vi "Execute.vi"(8 "error in (no error)":errorcluster, 10 "System In":refnum<class "abs_System.lvclass">, 11 "Node in":refnum<class "Set Boolean.lvclass">) -> (0 "error out":errorcluster, 1 "Status":T1, 2 "System Out":refnum<class "abs_System.lvclass">, 3 "Node out":refnum<class "Set Boolean.lvclass">)   [LabVIEW 2021, in "BT.lvlib" / "Set Boolean.lvclass"]
uses:
  Set Boolean.lvclass
  C:/Users/Tim/Documents/GitHub/LV_Behaviour_Tree/Source/abs_Type Leaf/abs_Type Leaf.lvclass
  abs_Node/Status.ctl
  abs_System/abs_System.lvclass
  LV_Abstract/Source/Abs_Types/Boolean/Abs_Boolean.lvclass
  C:/Users/Tim/Documents/GitHub/LV_Abstract/Source/Abs_Types/Type/Abs_Type.lvclass
  abs_Type Leaf/abs_Type Leaf.lvclass/abs_Type Leaf.ctl
  Set Boolean.lvclass/Set Boolean.ctl
  abs_Type Leaf/Properties/Read Value Class.vi
  Properties/Read Boolean.vi
  abs_Type Leaf/Properties/Write Value Class.vi
  LV_Abstract/Source/Abs_Types/Type/Abs_Type.lvclass
  abs_Type Leaf/abs_Type Leaf.lvclass
  abs_Node/abs_Node.lvclass
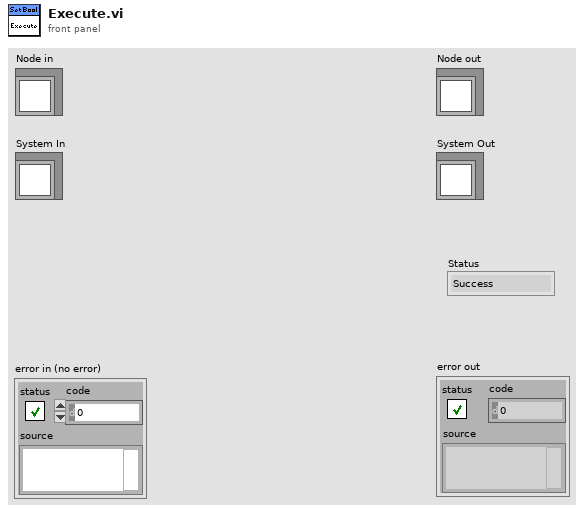
[diagram p1: front panel]
types:
  T1 = typedef "BT.lvlib/abs_Node.lvclass/Status.ctl" = enum16{"Success", "Failure", "Running"}
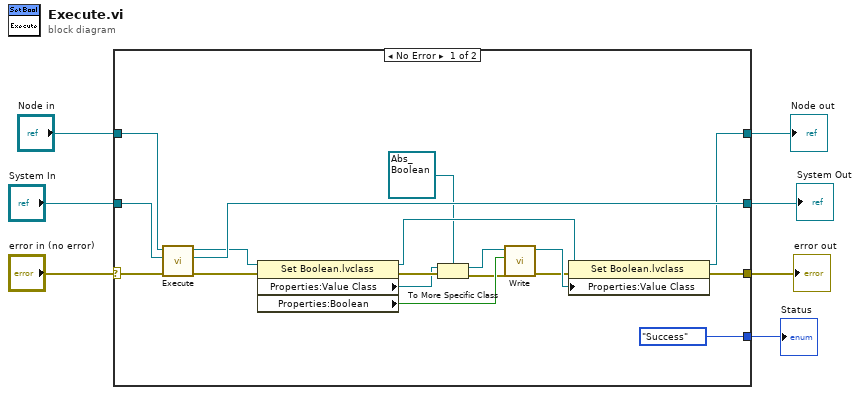
[diagram p0: block diagram]
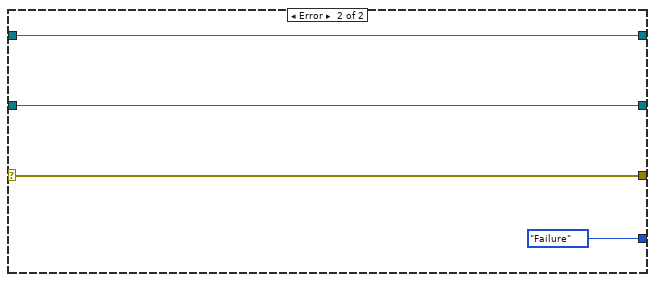
[diagram p2: hidden frame]
diagram:
  n1 = case shown="No Error" "error in (no error)" {
    selector: "error in (no error)" -> [w24 w27]
    tunnel: [w25 w28] -> w3
    tunnel: "System In" -> [w23 w28]
    tunnel: "Node in" -> [w22 w29]
    tunnel: [w18 w27] -> w4
    tunnel: [w17 w29] -> w2
    tunnel: [Status."Success" ("Status") Status."Failure" ("Status")] -> w1
    frame No Error {
      n2 = call-parent "Execute.vi"("error in (no error)"=w24, "System In"=w23, "Node in"=w22) -> ("error out"=w21:errorcluster, "System Out"=w25:refnum<class "abs_System.lvclass">, "Node out"=w20:refnum<class "Set Boolean.lvclass">)  [unwired: 5 in, 1 out]
      n3 = property class="Set Boolean.lvclass"(reference=w20, error in=w21) -> (reference out=w19:refnum<class "Set Boolean.lvclass">, error out=w12:errorcluster, "Properties:Value Class"=w11:refnum<class "Abs_Type.lvclass">, "Properties:Boolean"=w13:bool)
      n4 = To More Specific Class(target class=refnum<class "Abs_Boolean.lvclass"> refnum ("Boolean in"), reference=w11, error in=w12) -> (specific class reference=w8:refnum<class "Abs_Boolean.lvclass">, error out=w10:errorcluster)
      n5 = call-dynamic "Write.vi"("error in (no error)"=w10, "Boolean"=w13, "Boolean in"=w8) -> ("error out"=w14:errorcluster, "Boolean out"=w15:refnum<class "Abs_Boolean.lvclass">)  [unwired: 7 in]
      n6 = property class="Set Boolean.lvclass"(reference=w19, error in=w14, "Properties:Value Class"=w15) -> (reference out=w17:refnum<class "Set Boolean.lvclass">, error out=w18:errorcluster)
    }
    frame Error {
    }
  }
  "error out" <- w4
  "Node out" <- w2
  "Status" <- w1
  "System Out" <- w3
